vi "get log folder path.vi"() -> (0 "log folder path":path)   [LabVIEW 2020, in "app_log.lvlib"]
uses:
  app_log.lvlib
  main/main.lvlib
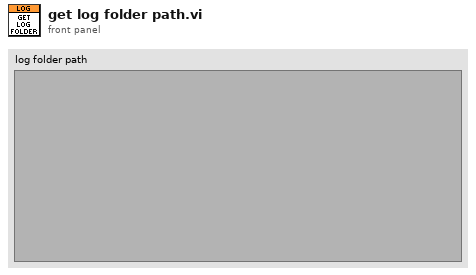
[diagram p1: front panel]
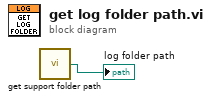
[diagram p0: block diagram]
diagram:
  n1 = call "get support folder path.vi"() -> ("support folder path"=→"log folder path":path)
